vi "SECS Receive.vi"(8 "error in (no error)":errorcluster, 10 "SECS-II Class":refnum<class "SECS-II Class.lvclass">, 11 "Scenarios Class in":refnum<class "Scenarios Class.lvclass">) -> (0 "error out":errorcluster, 3 "Scenarios Class out":refnum<class "Scenarios Class.lvclass">)   [LabVIEW 2020, in "SECS Scenarios.lvlib" / "Scenarios Class.lvclass"]
uses:
  Scenarios Class.lvclass
  SECS Communication/SECS-II Class/SECS-II Class.lvclass
  01-Establish Communications/01-Establish Communications.lvclass
  D:/Dropbox/SECS/SECS_GEM v1.1.0/Com/SECS Scenarios/Scenarios Class/Scenarios Class.lvclass
  02-Host Requests Status Variable Namelist/02-Host Requests Status Variable Namelist.lvclass
  03-Host Requests Current Status Variable Value/03-Host Requests Current Status Variable Value.lvclass
  04-Host Requests Equipment Current Constant Values/04-Host Requests Equipment Current Constant Values.lvclass
  05-Host Send Equipment Constant Values/05-Host Send Equipment Constant Values.lvclass
  06-Host Requests Status Equipment Constant Namelist/06-Host Requests Status Equipment Constant Namelist.lvclass
  08-Host Requsts Event Report/08-Host Requsts Event Report.lvclass
  09-Host Requsts Individual Report/09-Host Requsts Individual Report.lvclass
  10-On-Line Identification/10-On-Line Identification.lvclass
  12-Upload Alarm Information/12-Upload Alarm Information.lvclass
  13-EnableDisable Alarm/13-EnableDisable Alarm.lvclass
  15-Process Program Request/15-Process Program Request.lvclass
  16-Process Program Send/16-Process Program Send.lvclass
  17-Deleting a Process Program by Host/17-Deleting a Process Program by Host.lvclass
  18-Host Requests Equipment Process Program Directory/18-Host Requests Equipment Process Program Directory.lvclass
  19-Equipment Process Program Uploading/19-Equipment Process Program Uploading.lvclass
  20-Process Program Downloading/20-Process Program Downloading.lvclass
  22-Host Sends Information to Equipment/22-Host Sends Information to Equipment.lvclass
  26-Host Requests to Enter OFF-Line/26-Host Requests to Enter OFF-Line.lvclass
  27-Host Requests to Enter On-Line/27-Host Requests to Enter On-Line.lvclass
  28-Remote Control/28-Remote Control.lvclass
  30-Host Requests Equipment to Set Time/30-Host Requests Equipment to Set Time.lvclass
  31-Host Requests Time Value from Equipment/31-Host Requests Time Value from Equipment.lvclass
  32-Trace Data Collection/32-Trace Data Collection.lvclass
  33-RPTID Setup/33-RPTID Setup.lvclass
  34-CEID Setup/34-CEID Setup.lvclass
  35-CEID EnableDisable/35-CEID EnableDisable.lvclass
  36-List Enabled Alarm Data/36-List Enabled Alarm Data.lvclass
  Scenarios Class.lvclass/Scenarios Class.ctl
  Read HSMS Class.vi
  Read On-Line Notifier.vi
  Write HSMS Class.vi
  Write On-Line Notifier.vi
  SECS Communication/HSMS Class/HSMS Class.lvclass
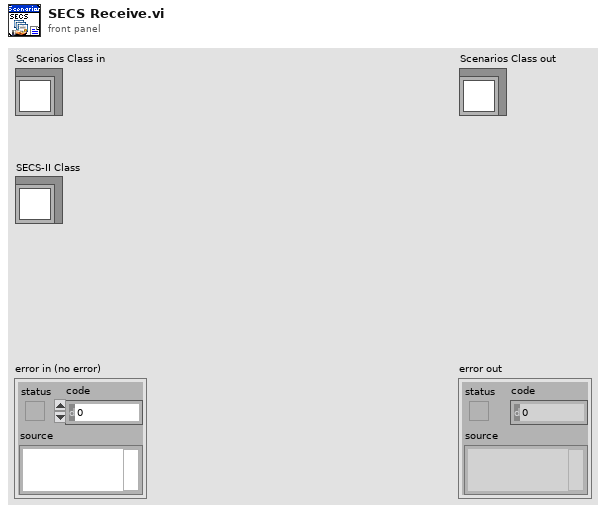
[diagram p1: front panel]
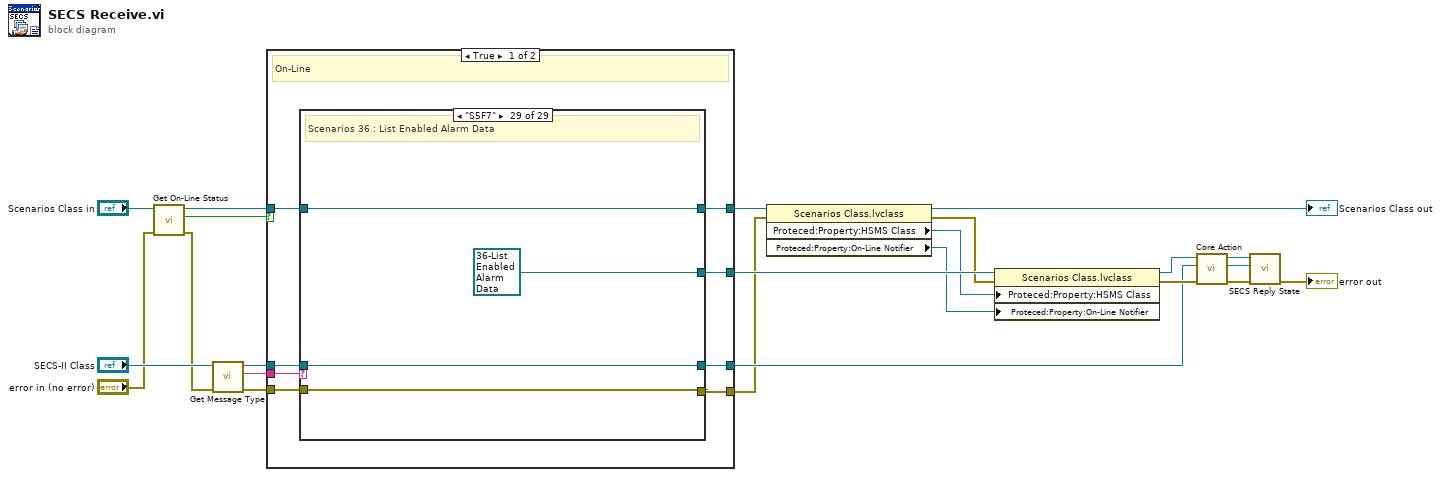
[diagram p0: block diagram]
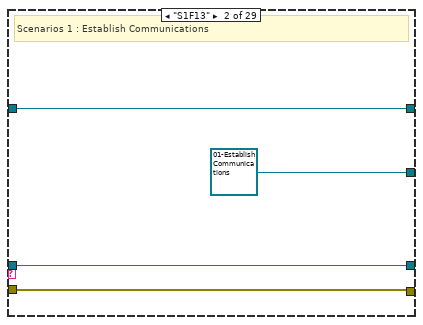
[diagram p3: hidden frame]
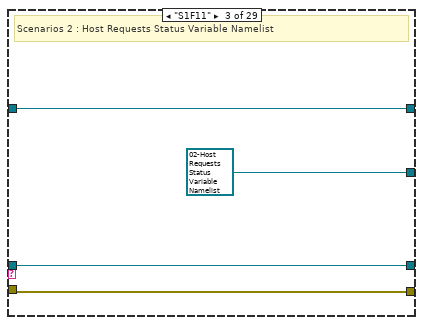
[diagram p4: hidden frame]
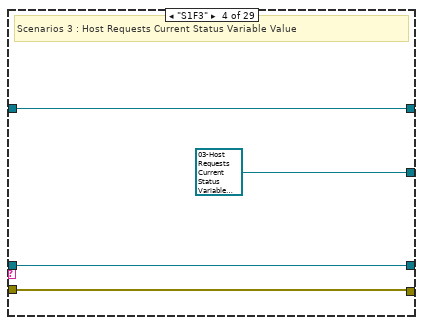
[diagram p5: hidden frame]
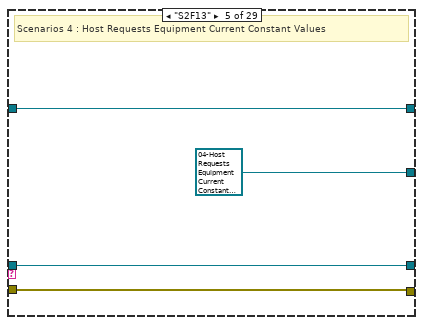
[diagram p6: hidden frame]
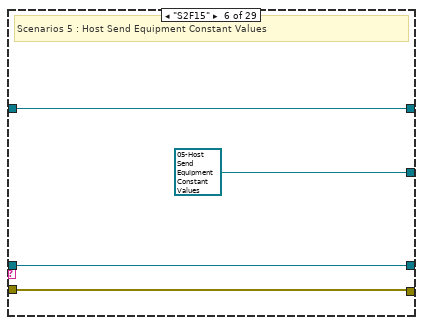
[diagram p7: hidden frame]
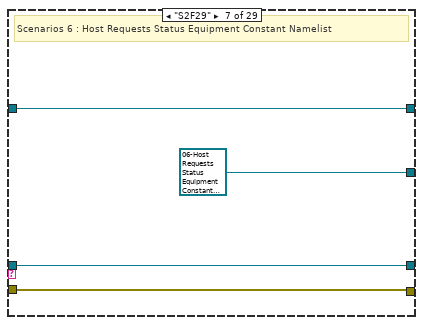
[diagram p8: hidden frame]
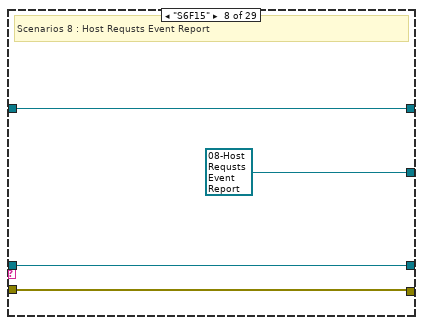
[diagram p9: hidden frame]
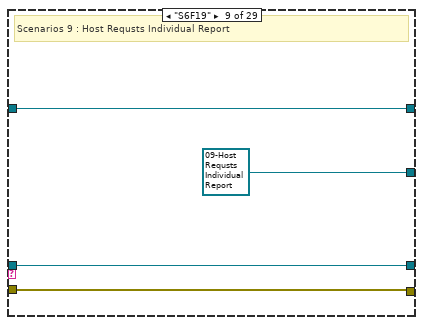
[diagram p10: hidden frame]
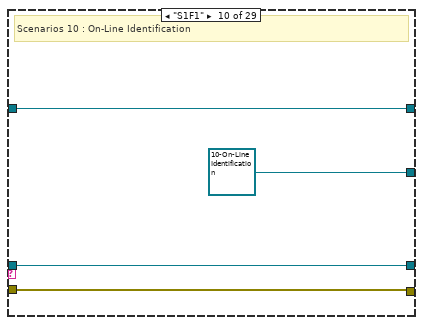
[diagram p11: hidden frame]
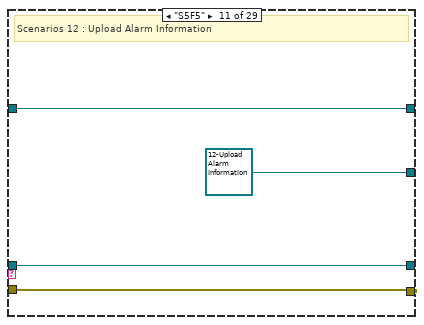
[diagram p12: hidden frame]
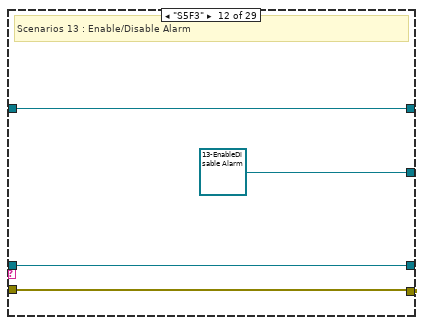
[diagram p13: hidden frame]
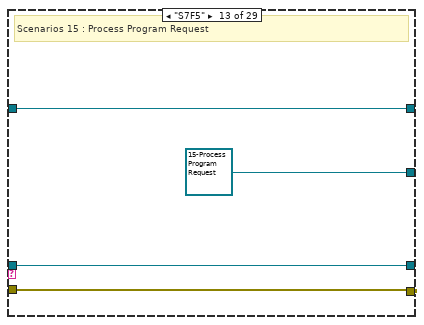
[diagram p14: hidden frame]
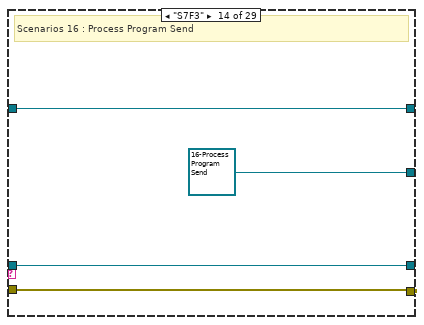
[diagram p15: hidden frame]
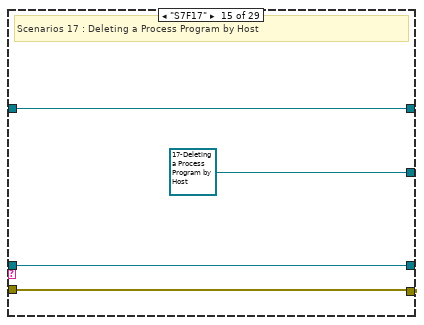
[diagram p16: hidden frame]
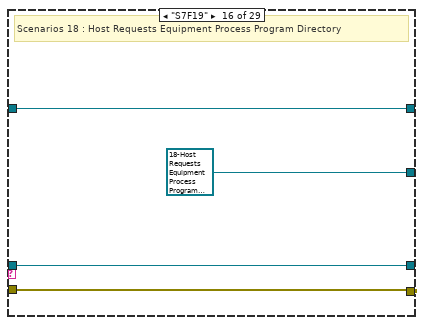
[diagram p17: hidden frame]
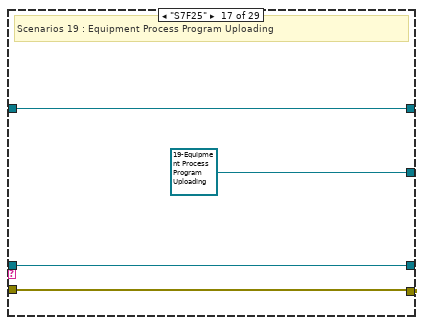
[diagram p18: hidden frame]
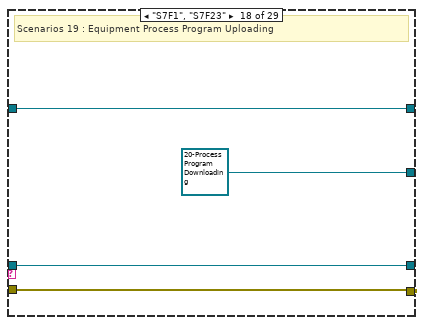
[diagram p19: hidden frame]
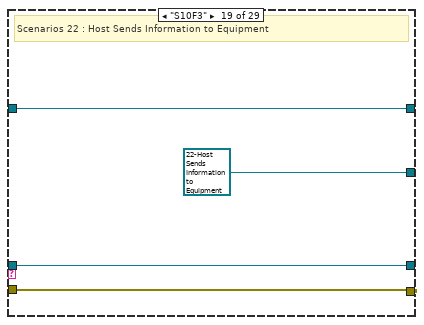
[diagram p20: hidden frame]
diagram:
  n1 = call "Get On-Line Status.vi"("error in (no error)"="error in (no error)", "Scenarios Class in"="Scenarios Class in") -> ("error out"=w3:errorcluster, "On-Line"=w2:bool, "Scenarios Class out"=w4:refnum<class "Scenarios Class.lvclass">)  [unwired: 7 in]
  n2 = call "Get Message Type.vi"("error in (no error)"=w3, "SECS-II Class in"="SECS-II Class") -> ("error out"=w23:errorcluster, "Message Type"=w22:string, "SECS-II Class out"=w21:refnum<class "SECS-II Class.lvclass">)  [unwired: 6 in, 1 out]
  n3 = case shown="True" w2 {
    tunnel: w23 -> [w31 w154]
    tunnel: w22 -> [w30 w153]
    tunnel: w21 -> [w29 w152]
    tunnel: [w28 w151] -> w17
    tunnel: [w27 w150] -> w16
    tunnel: [w26 w149] -> w13
    tunnel: [w25 w148] -> w12
    tunnel: w4 -> [w24 w147]
    frame True {
      # "On-Line"
      n4 = case shown="\"S5F7\"" w30 {
        tunnel: w31 -> [w34 w36 w41 w43 w49 w53 w57 w61 w65 w69 w73 w77 w81 w85 w89 w93 w97 w101 w105 w109 w113 w117 w121 w125 w129 w133 w137 w141 w145]
        tunnel: w29 -> [w33 w35 w40 w44 w48 w52 w56 w60 w64 w68 w72 w76 w80 w84 w88 w92 w96 w100 w104 w108 w112 w116 w120 w124 w128 w132 w136 w140 w144]
        tunnel: w24 -> [w32 w38 w42 w46 w50 w54 w58 w62 w66 w70 w74 w78 w82 w86 w90 w94 w98 w102 w106 w110 w114 w118 w122 w126 w130 w134 w138 w142 w146]
        tunnel: [w32 w38 w42 w46 w50 w54 w58 w62 w66 w70 w74 w78 w82 w86 w90 w94 w98 w102 w106 w110 w114 w118 w122 w126 w130 w134 w138 w142 w146] -> w27
        tunnel: [w34 w36 w41 w43 w49 w53 w57 w61 w65 w69 w73 w77 w81 w85 w89 w93 w97 w101 w105 w109 w113 w117 w121 w125 w129 w133 w137 w141 w145] -> w25
        tunnel: [w32 refnum<class "01-Establish Communications.lvclass"> refnum ("Establish Communications") refnum<class "02-Host Requests Status Variable Namelist.lvclass"> refnum ("SECS Bridge.lvlib:Host Requests Status Variable Namelist.lvclass") refnum<class "03-Host Requests Current Status Variable Value.lvclass"> refnum ("SECS Bridge.lvlib:Host Requests Current Status Variable Value.lvclass") refnum<class "04-Host Requests Equipment Current Constant Values.lvclass"> refnum ("SECS Bridge.lvlib:Host Requests Equipment Current Constant Values.lvclass") refnum<class "05-Host Send Equipment Constant Values.lvclass"> refnum ("SECS Scenarios.lvlib:05-Host Send Equipment Constant Values.lvclass") refnum<class "06-Host Requests Status Equipment Constant Namelist.lvclass"> refnum ("SECS Scenarios.lvlib:06-Host Requests Status Equipment Constant Namelist.lvclass") refnum<class "08-Host Requsts Event Report.lvclass"> refnum ("SECS Scenarios.lvlib:08-Host Requsts Event Report.lvclass") refnum<class "09-Host Requsts Individual Report.lvclass"> refnum ("SECS Scenarios.lvlib:09-Host Requsts Individual Report.lvclass") refnum<class "10-On-Line Identification.lvclass"> refnum ("SECS Scenarios.lvlib:10-On-Line Identification.lvclass") refnum<class "12-Upload Alarm Information.lvclass"> refnum ("SECS Scenarios.lvlib:12-Upload Alarm Information.lvclass") refnum<class "13-EnableDisable Alarm.lvclass"> refnum ("SECS Scenarios.lvlib:13-EnableDisable Alarm.lvclass") refnum<class "15-Process Program Request.lvclass"> refnum ("SECS Scenarios.lvlib:15-Process Program Request.lvclass") refnum<class "16-Process Program Send.lvclass"> refnum ("SECS Scenarios.lvlib:16-Process Program Send.lvclass") refnum<class "17-Deleting a Process Program by Host.lvclass"> refnum ("SECS Scenarios.lvlib:17-Deleting a Process Program by Host.lvclass") refnum<class "18-Host Requests Equipment Process Program Directory.lvclass"> refnum ("SECS Scenarios.lvlib:18-Host Requests Equipment Process Program Directory.lvclass") refnum<class "19-Equipment Process Program Uploading.lvclass"> refnum ("SECS Scenarios.lvlib:19-Equipment Process Program Uploading.lvclass") refnum<class "20-Process Program Downloading.lvclass"> refnum ("SECS Scenarios.lvlib:20-Process Program Downloading.lvclass") refnum<class "22-Host Sends Information to Equipment.lvclass"> refnum ("SECS Scenarios.lvlib:22-Host Sends Information to Equipment.lvclass") refnum<class "26-Host Requests to Enter OFF-Line.lvclass"> refnum ("SECS Scenarios.lvlib:26-Host Requests to Enter OFF-Line.lvclass") refnum<class "27-Host Requests to Enter On-Line.lvclass"> refnum ("SECS Scenarios.lvlib:27-Host Requests to Enter On-Line.lvclass") refnum<class "28-Remote Control.lvclass"> refnum ("SECS Scenarios.lvlib:28-Remote Control.lvclass") refnum<class "30-Host Requests Equipment to Set Time.lvclass"> refnum ("SECS Scenarios.lvlib:30-Host Requests Equipment to Set Time.lvclass") refnum<class "31-Host Requests Time Value from Equipment.lvclass"> refnum ("SECS Scenarios.lvlib:31-Host Requests Time Value from Equipment.lvclass") refnum<class "32-Trace Data Collection.lvclass"> refnum ("SECS Scenarios.lvlib:32-Trace Data Collection.lvclass") refnum<class "33-RPTID Setup.lvclass"> refnum ("SECS Scenarios.lvlib:33-RPTID Setup.lvclass") refnum<class "34-CEID Setup.lvclass"> refnum ("SECS Scenarios.lvlib:34-CEID Setup.lvclass") refnum<class "35-CEID EnableDisable.lvclass"> refnum ("SECS Scenarios.lvlib:35-CEID EnableDisable.lvclass") refnum<class "36-List Enabled Alarm Data.lvclass"> refnum ("SECS Scenarios.lvlib:36-List Enabled Alarm Data.lvclass")] -> w28
        tunnel: [w33 w35 w40 w44 w48 w52 w56 w60 w64 w68 w72 w76 w80 w84 w88 w92 w96 w100 w104 w108 w112 w116 w120 w124 w128 w132 w136 w140 w144] -> w26
        frame Default {
          # "Message fault due to Unrecognized Stream Type\nMessage fault due to Unrecognized Function Type"
        }
        frame "S1F13" {
          # "Scenarios 1 : Establish Communications"
        }
        frame "S1F11" {
          # "Scenarios 2 : Host Requests Status Variable Namelist"
        }
        frame "S1F3" {
          # "Scenarios 3 : Host Requests Current Status Variable Value"
        }
        frame "S2F13" {
          # "Scenarios 4 : Host Requests Equipment Current Constant Values"
        }
        frame "S2F15" {
          # "Scenarios 5 : Host Send Equipment Constant Values"
        }
        frame "S2F29" {
          # "Scenarios 6 : Host Requests Status Equipment Constant Namelist"
        }
        frame "S6F15" {
          # "Scenarios 8 : Host Requsts Event Report"
        }
        frame "S6F19" {
          # "Scenarios 9 : Host Requsts Individual Report"
        }
        frame "S1F1" {
          # "Scenarios 10 : On-Line Identification"
        }
        frame "S5F5" {
          # "Scenarios 12 : Upload Alarm Information"
        }
        frame "S5F3" {
          # "Scenarios 13 : Enable/Disable Alarm"
        }
        frame "S7F5" {
          # "Scenarios 15 : Process Program Request"
        }
        frame "S7F3" {
          # "Scenarios 16 : Process Program Send"
        }
        frame "S7F17" {
          # "Scenarios 17 : Deleting a Process Program by Host"
        }
        frame "S7F19" {
          # "Scenarios 18 : Host Requests Equipment Process Program Directory"
        }
        frame "S7F25" {
          # "Scenarios 19 : Equipment Process Program Uploading"
        }
        frame "S7F1", "S7F23" {
          # "Scenarios 19 : Equipment Process Program Uploading"
        }
        frame "S10F3" {
          # "Scenarios 22 : Host Sends Information to Equipment"
        }
        frame "S1F15" {
          # "Scenarios 26 : Host Requests to Enter OFF-Line"
        }
        frame "S1F17" {
          # "Scenarios 27 : Host Requests to Enter On-Line"
        }
        frame "S2F41" {
          # "Scenarios 28 : Remote Control"
        }
        frame "S2F31" {
          # "Scenarios 30 : Host Requests Equipment to Set Time"
        }
        frame "S2F17" {
          # "Scenarios 31 : Host Requests Time Value from Equipment"
        }
        frame "S2F23" {
          # "Scenarios 32 : Trace Data Collection"
        }
        frame "S2F33" {
          # "Scenarios 33 : RPTID Setup"
        }
        frame "S2F35" {
          # "Scenarios 34 : CEID Setup"
        }
        frame "S2F37" {
          # "Scenarios 35 : CEID Enable/Disable"
        }
        frame "S5F7" {
          # "Scenarios 36 : List Enabled Alarm Data"
        }
      }
    }
    frame False {
      # "Off-Line 只接受S1F13、S1F17"
      n5 = case shown="\"S1F13\"" w153 {
        tunnel: w154 -> [w155 w159 w164]
        tunnel: w152 -> [w157 w158 w163]
        tunnel: w147 -> [w156 w161 w165]
        tunnel: [w156 w161 w165] -> w150
        tunnel: [w155 w159 w164] -> w148
        tunnel: [w156 refnum<class "01-Establish Communications.lvclass"> refnum ("Establish Communications") refnum<class "27-Host Requests to Enter On-Line.lvclass"> refnum ("SECS Scenarios.lvlib:27-Host Requests to Enter On-Line.lvclass")] -> w151
        tunnel: [w157 w158 w163] -> w149
        frame Default {
        }
        frame "S1F13" {
          # "Scenarios 1 : Establish Communications"
        }
        frame "S1F17" {
          # "Scenarios 27 : Host Requests to Enter On-Line"
        }
      }
    }
  }
  n6 = property class="Scenarios Class.lvclass"(reference=w16, error in=w12) -> (reference out=→"Scenarios Class out":refnum<class "Scenarios Class.lvclass">, error out=w14:errorcluster, "Proteced:Property:HSMS Class"=w15:refnum<class "HSMS Class.lvclass">, "Proteced:Property:On-Line Notifier"=w6:refnum<notifier>)
  n7 = property class="Scenarios Class.lvclass"(reference=w17, error in=w14, "Proteced:Property:HSMS Class"=w15, "Proteced:Property:On-Line Notifier"=w6) -> (reference out=w19:refnum<class "Scenarios Class.lvclass">, error out=w18:errorcluster)
  n8 = call-dynamic "Core Action.vi"("error in (no error)"=w18, "SECS-II Class In"=w13, "Scenarios Class in"=w19) -> ("error out"=w10:errorcluster, "SECS-II Class Out"=w7:refnum<class "SECS-II Class.lvclass">, "Scenarios Class out"=w9:refnum<class "Scenarios Class.lvclass">)  [unwired: 6 in]
  n9 = call "SECS Reply State.vi"("error in (no error)"=w10, "SECS-II Class In"=w7, "Scenarios Class in"=w9) -> ("error out"=→"error out":errorcluster)  [unwired: 7 in, 1 out]
